vi "Quench_CalcR(SubVI).vi"(0 "Mag":fxp<+,16,14>, 5 "input valid":bool, 9 "count done?":bool) -> ()   [LabVIEW 2018]
uses:
  <vilib>/rvi/FXPMathLib/FxpDiv/subVIs/nifxpmath_Div_SimConfig.ctl
  <vilib>/rvi/FXPMathLib/FxpDiv/simVIs/DllFxpDivTemp_sub.vi
  <vilib>/rvi/Emulation/niFpgaEmulationIsFPGAContextNoSignature.vi
  <vilib>/rvi/DataTransferAndStorage/Container/Common/niFpgaContainerGetUniqueNameForEmu.vi
  <vilib>/rvi/Memory/Memory_Emulation/niFpgaMemoryEmulationCacheClearOnFirstRun.vi
  <vilib>/rvi/Memory/Memory_Emulation/nirvimemoryEmulationManagerCache_MakeExclusive.vi
  <vilib>/rvi/Memory/Memory_Emulation/niFpgaMemoryEmulationValidateCache.vi
  <vilib>/rvi/Memory/Memory_Emulation/nirvimemoryEmulationManagerCache_InsertValue.vi
  <vilib>/Utility/error.llb/Clear Errors.vi
  <vilib>/rvi/Memory/Memory_Emulation/nirvimemoryEmulationManagerCache_ReleaseExclusive.vi
  <vilib>/rvi/Memory/Memory_Emulation/nirvimemoryEmulationManagerCache_GetValue.vi
  <vilib>/rvi/Memory/Memory_Emulation/nirvimemoryEmulationManagerCache_SetValue.vi
  <vilib>/rvi/Emulation/niFpgaProcessEmulError.vi
  <vilib>/rvi/Emulation/niFpgaSctlEmulationGetInTimedLoop.vi
  <vilib>/rvi/FXPMathLib/FxpSub/XNode/nifxpmath_Sub.xnode
  <vilib>/rvi/FXPMathLib/FxpInterpret/XNode/nifxpmath_Interpret.xnode
  <vilib>/rvi/FXPMathLib/FxpDiv/XNode/nifxpmath_Div.xnode
  <vilib>/rvi/DataTransferAndStorage/Container/XNode/niFpgaContainer.xnode
  <vilib>/rvi/DataTransferAndStorage/Register/Emulation/niFpgaRegisterEmulation.vi
  <vilib>/rvi/FXPMathLib/sim/FxpSim.dll
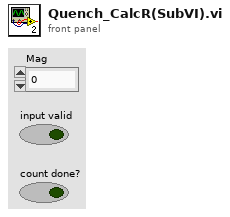
[diagram p1: front panel]
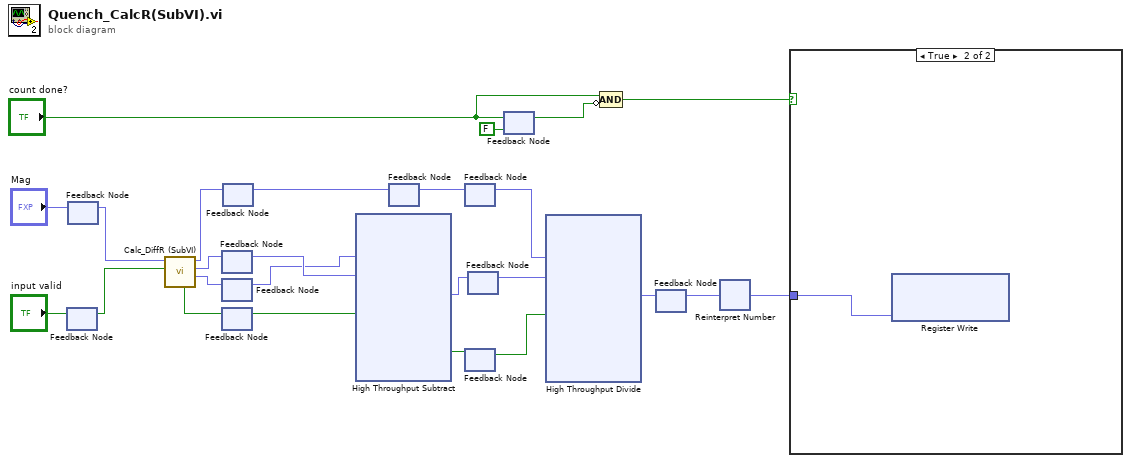
[diagram p0: block diagram]
diagram:
  n1 = feedback #1() -> (w17:bool)  [unwired: 1 in]
  n2 = feedback-in #1("input valid") -> ()
  n3 = feedback #2() -> (w16:fxp<+,16,14>)  [unwired: 1 in]
  n4 = feedback-in #2("Mag") -> ()
  n5 = call "Calc_DiffR (SubVI).vi"("input valid in"=w17, "Mag 3"=w16) -> ("Mag 1"=w13:fxp<+,16,14>, "Mag 2"=w14:fxp<+,16,14>, "Mag 4"=w15:fxp<+,16,14>, "input valid out"=w12:bool)  [unwired: 6 in]
  n6 = feedback #3() -> (w3:fxp<+,16,14>)  [unwired: 1 in]
  n7 = feedback-in #3(w14) -> ()
  n8 = feedback #4() -> (w2:fxp<+,16,14>)  [unwired: 1 in]
  n9 = feedback-in #4(w13) -> ()
  n10 = feedback #5() -> (w11:bool)  [unwired: 1 in]
  n11 = feedback-in #5(w12) -> ()
  n12 = feedback #6() -> (w10:fxp<+,16,14>)  [unwired: 1 in]
  n13 = feedback-in #6(w15) -> ()
  n14 = xnode "High Throughput Subtract"("x"=w2, "y"=w3, "input valid"=w11) -> ("x-y"=w9:fxp<+/-,16,14>, "output valid"=w24:bool)  [unwired: 1 in, 1 out]
  n15 = feedback #7() -> (w22:fxp<+,16,14>)  [unwired: 1 in]
  n16 = feedback-in #7(w10) -> ()
  n17 = feedback #8() -> (w5:fxp<+,16,14>)  [unwired: 1 in]
  n18 = feedback-in #8(w22) -> ()
  n19 = feedback #9() -> (w4:bool)  [unwired: 1 in]
  n20 = feedback-in #9(w24) -> ()
  n21 = feedback #10() -> (w6:fxp<+/-,16,14>)  [unwired: 1 in]
  n22 = feedback-in #10(w9) -> ()
  n23 = feedback #11(FALSE ("count done?")) -> (w21:bool)
  n24 = feedback-in #11("count done?") -> ()
  n25 = xnode "High Throughput Divide"("x"=w5, "y"=w6, "input valid"=w4) -> ("x/y"=w7:fxp<+/-,32,18>)  [unwired: 1 in, 2 out]
  n26 = Compound Arithmetic op=AND("count done?", invert w21) -> (w18:bool)
  n27 = feedback #12() -> (w8:fxp<+/-,32,18>)  [unwired: 1 in]
  n28 = feedback-in #12(w7) -> ()
  n29 = xnode "Reinterpret Number"("x"=w8) -> ("y"=w1:fxp<+/-,32,13>)
  n30 = case shown="True" w18 {
    tunnel: w1 -> [_ w26]
    frame False {
    }
    frame True {
      n31 = xnode "Register Write"("Data"=w26) -> ()  [unwired: 1 in, 1 out]
    }
  }
